vi "IsDefault.vi"(1 "Address":u16) -> (0 "Default?":bool)   [LabVIEW 2010, in "FTC.lvlib" / "Remote Interface.lvlib"]
uses:
  Remote Interface.lvlib
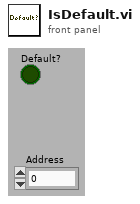
[diagram p1: front panel]
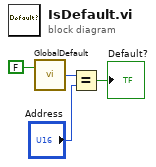
[diagram p0: block diagram]
diagram:
  n1 = call "GlobalDefault.vi"("Write?"=FALSE) -> ("Default"=w1:u16)  [unwired: 1 in]
  n2 = Equal?(x=w1, y="Address") -> (x = y?=→"Default?":bool)
